vi "GetCyclicDataTC110.vi"(8 "error in (no error)":errorcluster, 9 "Map":map{T1, variant}(c390), 10 "Adress of unit":u16, 11 "VISA Refnum in":refnum<visa-resource-name>) -> (0 "error out":errorcluster, 2 "Map 2":map{T1, variant}(c390), 3 "VISA session out":refnum<visa-resource-name>)   [LabVIEW 2019]
uses:
  PfeifferTC110Cmds.ctl
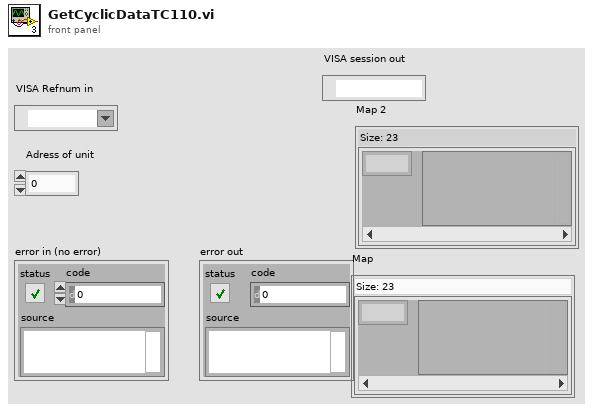
[diagram p1: front panel]
types:
  T1 = typedef "PfeifferTC110Cmds.ctl" = enum16{"Standby", "AckError", "Run", "Motor", "SpdSwPtAtt", "ErrorCode", "OvTempElec", "OvTempPump", "SetSpdAtt", "PumpAccel", "ActualSpdHz", "DrvCurrent", "OpHrsPump", "FwVersion", "DrvVoltage", "OpHrsElec", "NominalSpd", "DrvPower", "PumpCycles", "TempElec", "TempPmpBot", "AccelDecel", "TempBearing", "TempMotor", "ElecName", "HWVersion", "SetRotSpdRPM", "ActualSpdRPM", "NominalSpdRPM"}
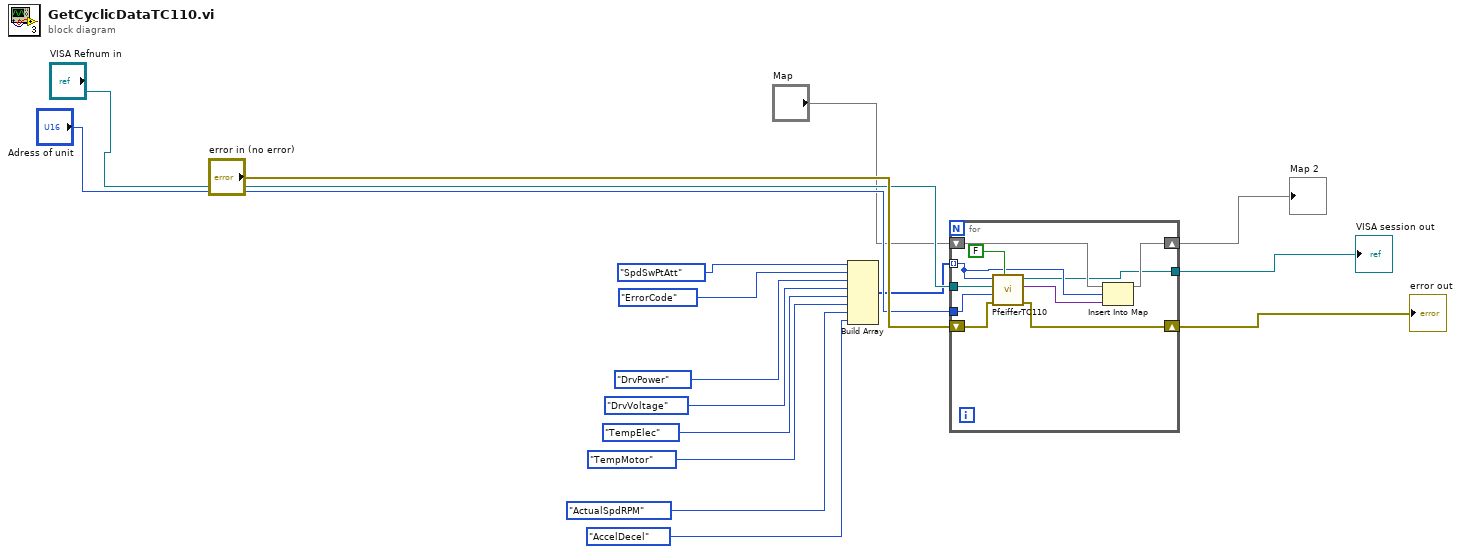
[diagram p0: block diagram]
diagram:
  n1 = Build Array(PfeifferTC110Cmds."SpdSwPtAtt" ("CMD ID"), PfeifferTC110Cmds."ErrorCode" ("CMD ID"), PfeifferTC110Cmds."DrvPower" ("CMD ID"), PfeifferTC110Cmds."DrvVoltage" ("CMD ID"), PfeifferTC110Cmds."TempElec" ("CMD ID"), PfeifferTC110Cmds."TempMotor" ("CMD ID"), PfeifferTC110Cmds."ActualSpdRPM" ("CMD ID"), PfeifferTC110Cmds."AccelDecel" ("CMD ID")) -> (w11:T1[])
  n2 = for {
    tunnel: w11 -> [w21] mode=indexing
    tunnel: "VISA Refnum in" -> [w25]
    tunnel: "Adress of unit" -> [w24]
    shift-right: [w22] -> w1
    shift-left: "Map" -> [w23]
    shift-right: [w19] -> w16
    shift-left: "error in (no error)" -> [w20]
    tunnel: [w17] -> w2
    n3 = call "PfeifferTC110.vi"("Write?"=FALSE, "error in"=w20, "Adress"=w24, "VISA session"=w25, "CMD ID"=w21) -> ("error out"=w19:errorcluster, "Response"=w18:variant, "VISA session out"=w17:refnum<visa-resource-name>)  [unwired: 4 in]
    n4 = Insert Into Map(map in=w23, key=w21, value=w18) -> (map out=w22:map{T1, variant})  [unwired: 2 out]
  }
  "error out" <- w16
  "VISA session out" <- w2
  "Map 2" <- w1
